vi "Setter Scripting.vi"(10 "Accessor Options":T1, 11 "VI Refnum":refnum<vi>) -> ()   [LabVIEW 2018, in "LVClassByRef.lvlib"]
uses:
  <resource>/Framework/Providers/LVClassByRef/LVClassByRef.lvlib
  <resource>/Framework/Providers/LVClassByRef/Accessor Options.ctl
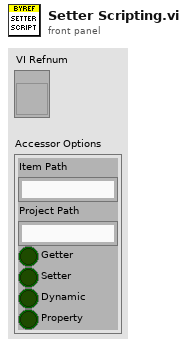
[diagram p1: front panel]
types:
  T1 = typedef "LVClassByRef.lvlib/Accessor Options.ctl" = cluster{"Item Path":string, "Project Path":string, "Getter":bool, "Setter":bool, "Dynamic":bool, "Property":bool}
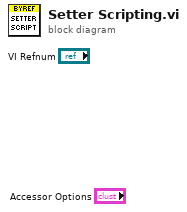
[diagram p0: block diagram]
diagram:
